vi "Open Build.vi"(8 "error in (no error)":errorcluster, 10 "Build specification name":string, 11 "TargetItem Refnum":refnum<vi>) -> (0 "error out":errorcluster, 3 "PPL out":refnum<class "NI_AB_API_DPPL.lvclass">)   [LabVIEW 2020, in "NI_AB_API_DPPL.lvclass"]
uses:
  <vilib>/AppBuilder/AB_API/DPPL/NI_AB_API_DPPL.lvclass
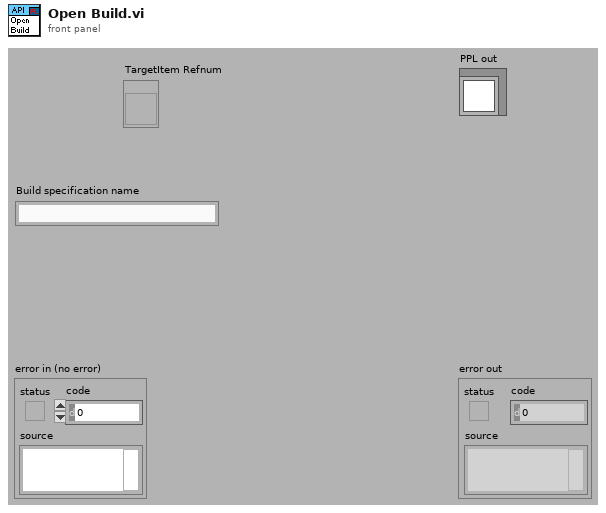
[diagram p1: front panel]
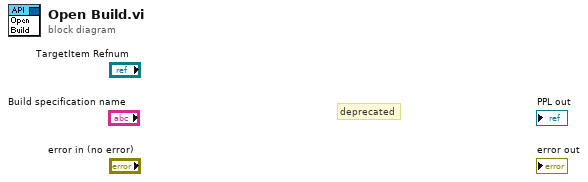
[diagram p0: block diagram]
diagram:
  # "deprecated"
